vi "Test UTF8 Compatibility in Report.vi"(8 "error in (no error)":errorcluster, 11 "Force FAIL?":bool) -> (0 "error out":errorcluster)   [LabVIEW 2020]
uses:
  classes/Test/Test.lvclass
  classes/Assert/Assert.lvclass
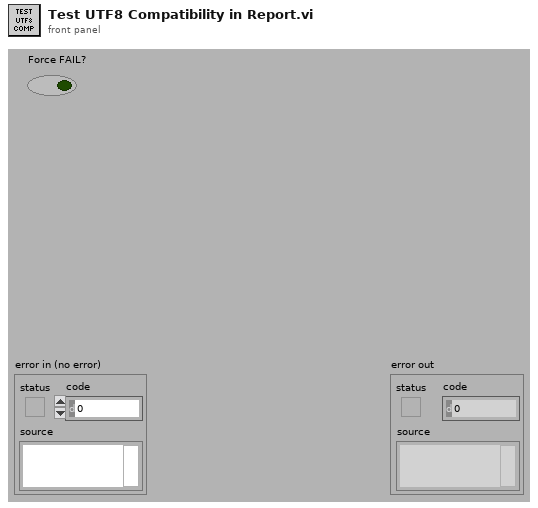
[diagram p1: front panel]
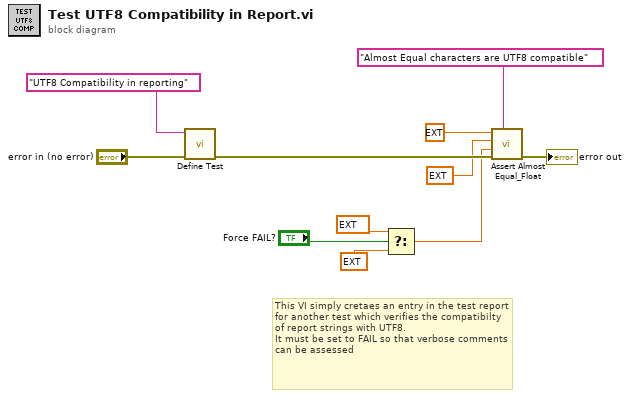
[diagram p0: block diagram]
diagram:
  # "This VI simply cretaes an entry in the test report for another test which verifies the compatibilty of report strings with UTF8.\nIt must be set to FAIL so that verbose comments can be assessed"
  n1 = call "Define Test.vi"("error in (no error)"="error in (no error)", "Label (VI Title)"="UTF8 Compatibility in reporting") -> ("error out"=w9:errorcluster)  [unwired: 8 in, 1 out]
  n2 = Select(t=ext 0.00099999999999999999996 ("X"), s="Force FAIL?", f=ext 0.02 ("X")) -> (s? t:f=w1:ext)
  n3 = call "Assert Almost Equal_Float.vi"("Label"="Almost Equal characters are UTF8 compatible" ("Label (VI Title)"), "error in (no error)"=w9, "Tolerance"=w1, "Y"=ext 1.01 ("X"), "X"=ext 1.0) -> ("error out"=→"error out":errorcluster)  [unwired: 5 in, 1 out]
